vi "FringeScannerOpenSynchronization.vi"(9 "error in (no error)":errorcluster) -> (2 "FringeTrackerSynchro":T1, 6 "error out":errorcluster)   [LabVIEW 2009]
uses:
  Controls/FringeTrackerSynchro.ctl
  Controls/FringeScannerCommand.ctl
  Controls/FringeScannerData.ctl
  Nicmos/Controls/NICMOS.READOUT.ctl
  Controls/FringeScannerState.ctl
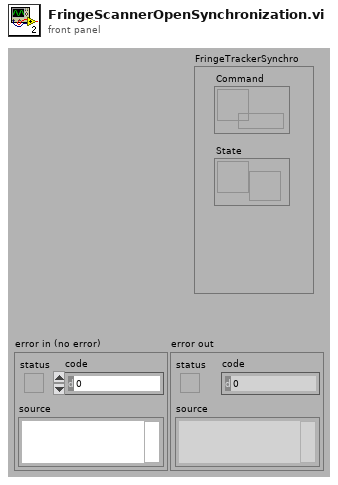
[diagram p1: front panel]
types:
  T1 = typedef "FringeTrackerSynchro.ctl" = cluster{"Command":refnum<queue>, "State":refnum<notifier>}
  T2 = typedef "FringeScannerState.ctl" = enum16{"IDLING", "CONFIGURING", "SCANNING", "STOPPING"}
  T3 = typedef "FringeScannerCommand.ctl" = cluster{"Command":enum16{"IDLE", "SCAN", "QUIT"}, "FringeScannerData":T4}
  T4 = typedef "FringeScannerData.ctl" = cluster{"Readout":T5, "Wavelength":dbl[unit], "Frame per fringe":dbl, "Autcollimation":bool}
  T5 = typedef "NICMOS.READOUT.ctl" = cluster{"Readout":i32, "Deglitch":i32, "Framerate":dbl[unit], "Bank":i32}
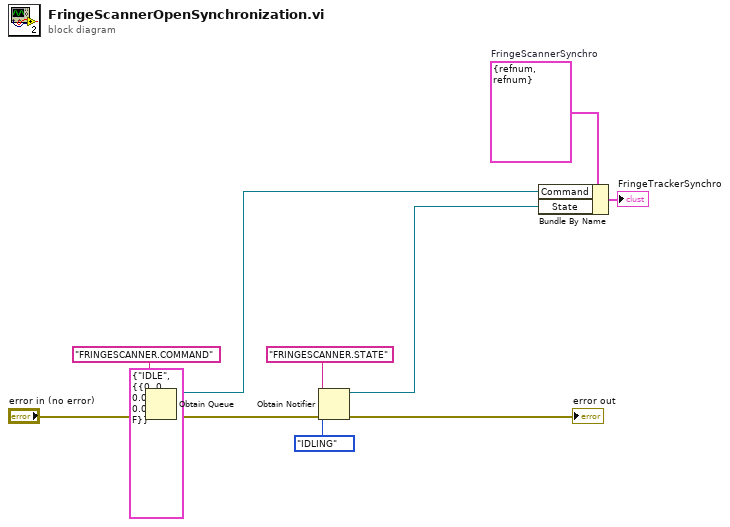
[diagram p0: block diagram]
diagram:
  w5 = T1 {"Command"=refnum, "State"=refnum}  # FringeScannerSynchro
  n1 = Obtain Queue(name (unnamed)="FRINGESCANNER.COMMAND", element data type=T3 {"Command"=enum."IDLE", "FringeScannerData"={"Readout"={"Readout"=0, "Deglitch"=0, "Framerate"=0.0, "Bank"=0}, "Wavelength"=0.0, "Frame per fringe"=0.0, "Autcollimation"=FALSE}} ("FringeScannerCommand"), error in (no error)="error in (no error)") -> (queue out=w4:refnum<queue>, error out=w8:errorcluster)  [unwired: 2 in, 1 out]
  n2 = Obtain Notifier(name (unnamed)="FRINGESCANNER.STATE", notification data type=FringeScannerState."IDLING" ("FringeScannerState"), error in (no error)=w8) -> (notifier out=w3:refnum<notifier>, error out=→"error out":errorcluster)  [unwired: 1 in, 1 out]
  n3 = Bundle By Name(cluster=w5, "Command"=w4, "State"=w3) -> (→"FringeTrackerSynchro":T1)
